vi "CloseConnection.vi"(0 "TCP Socket in":refnum<class "Socket Communication.lvclass">, 5 "error in (no error)":errorcluster) -> (14 "TCP Socket out":refnum<class "Socket Communication.lvclass">, 19 "error out":errorcluster)   [LabVIEW 2016, in "Socket Communication.lvclass"]
uses:
  Socket Communication.lvclass
  Socket Communication.lvclass/Socket Communication.ctl
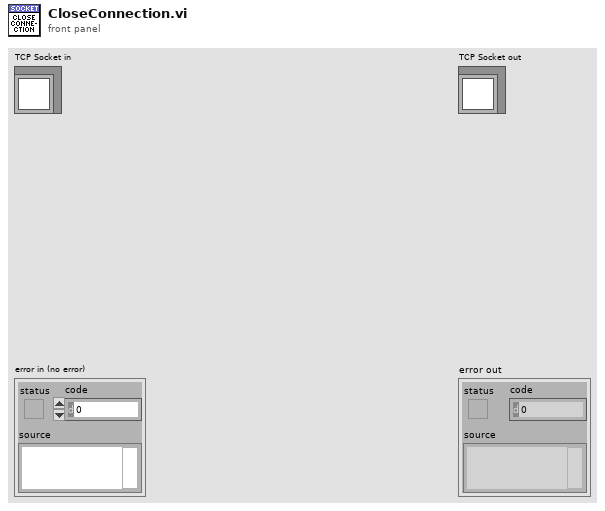
[diagram p1: front panel]
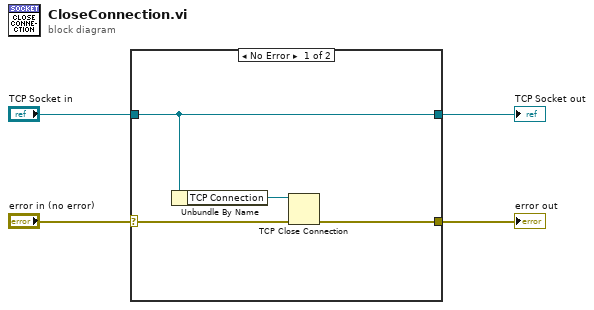
[diagram p0: block diagram]
diagram:
  n1 = case shown="No Error" "error in (no error)" {
    selector: "error in (no error)" -> [w7 w10]
    tunnel: [w5 w10] -> w3
    tunnel: [w8 w9] -> w1
    tunnel: "TCP Socket in" -> [w8 w9]
    frame No Error {
      n2 = Unbundle By Name(w8) -> ("TCP Connection"=w6:refnum<k5>)
      n3 = TCP Close Connection(connection ID=w6, error in (no error)=w7) -> (error out=w5:errorcluster)  [unwired: 1 in, 1 out]
    }
    frame Error {
    }
  }
  "error out" <- w3
  "TCP Socket out" <- w1
